vi "ClimbSequencer.vi"(7 "Reinit":bool) -> (0 "Climber Climbing":bool, 1 "Climber Power":dbl, 2 "Climber Pin":bool, 3 "PTO":bool)   [LabVIEW 2019]
doc: "This VI contains the endgame climb sequencer."
uses:
  dscommands.vi
  78443452-49a0-4252-95b8-0a958b59513b.vi
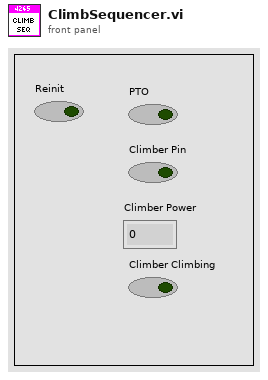
[diagram p1: front panel]
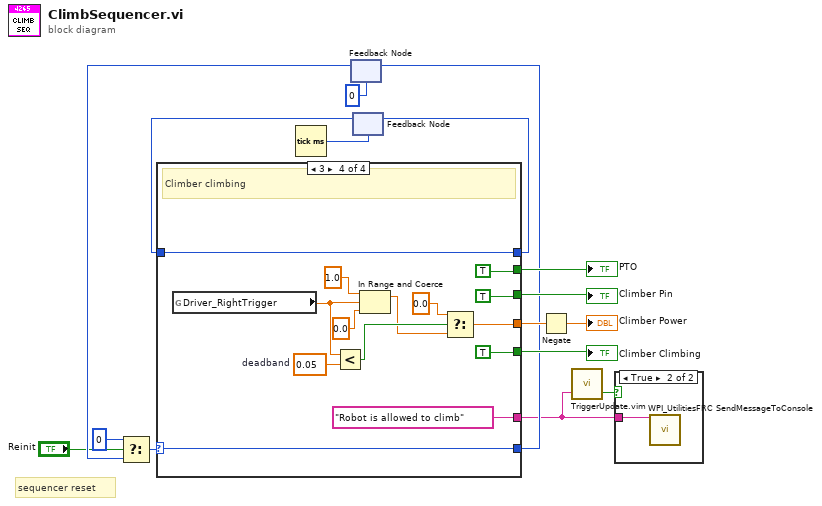
[diagram p0: block diagram]
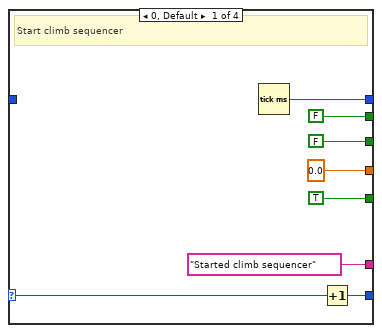
[diagram p3: hidden frame]
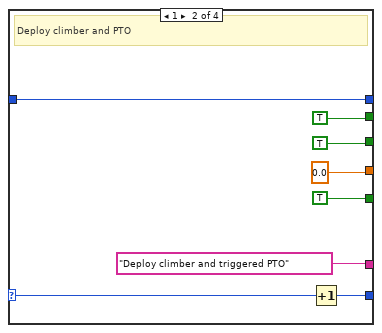
[diagram p4: hidden frame]
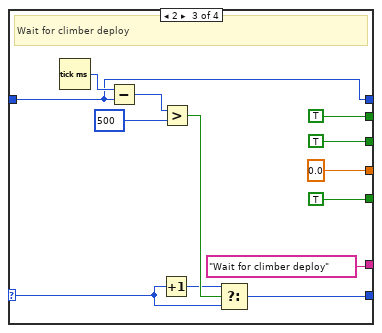
[diagram p5: hidden frame]
diagram:
  # "sequencer reset"
  n1 = Tick Count (ms)() -> (millisecond timer value=w7:u32)
  n2 = feedback #1(0) -> (w13:i32)
  n3 = Select(t=0, s="Reinit", f=w13) -> (s? t:f=w15:i32)
  n4 = feedback #2(w7) -> (w6:u32)
  n5 = case shown="3" w15 {
    selector: w15 -> [w22 w32 w41 w58]
    tunnel: [w21 w27 w39 w58] -> w3
    tunnel: ["Started climb sequencer" "Deploy climber and triggered PTO" "Wait for climber deploy" "Robot is allowed to climb"] -> w2
    tunnel: [w24 w28 w38 w57] -> w5
    tunnel: w6 -> [_ w28 w38 w57]
    tunnel: [0.0 ("Climber_Power") 0.0 ("Climber_Power") 0.0 ("Climber_Power") w53] -> w8
    tunnel: [FALSE TRUE TRUE TRUE] -> w9
    tunnel: [FALSE TRUE TRUE TRUE] -> w10
    tunnel: [TRUE TRUE TRUE TRUE] -> w11
    frame 0, Default {
      # "Start climb sequencer"
      n6 = Tick Count (ms)() -> (millisecond timer value=w24:u32)
      n7 = Increment(x=w22) -> (x+1=w21:i32)
    }
    frame 1 {
      # "Deploy climber and PTO"
      n8 = Increment(x=w32) -> (x+1=w27:i32)
    }
    frame 2 {
      # "Wait for climber deploy"
      n9 = Tick Count (ms)() -> (millisecond timer value=w45:u32)
      n10 = Subtract(x=w45, y=w38) -> (x-y=w44:u32)
      n11 = Increment(x=w41) -> (x+1=w40:i32)
      n12 = Greater?(x=w44, y=u32 500) -> (0:w42:bool)
      n13 = Select(t=w40, s=w42, f=w41) -> (s? t:f=w39:i32)
    }
    frame 3 {
      w50 = 0.05  # deadband
      # "Climber climbing"
      n14 = global read "dscommands.vi" "Driver_RightTrigger"() -> (w46:dbl)
      n15 = Less?(x=w46, y=w50) -> (x < y?=w52:bool)
      n16 = In Range and Coerce(upper limit=1.0, x=w46, lower limit=0.0) -> (coerced(x)=w49:dbl)  [unwired: 1 out]
      n17 = Select(t=0.0, s=w52, f=w49) -> (s? t:f=w53:dbl)
    }
  }
  "Climber Climbing" <- w11
  "Climber Pin" <- w10
  "PTO" <- w9
  n18 = feedback-in #1(w3) -> ()
  n19 = feedback-in #2(w5) -> ()
  n20 = Negate(x=w8) -> (-x=→"Climber Power":dbl)
  n21 = call "TriggerUpdate.vim"("Trigger"=w2) -> ("Update"=w1:bool)  [unwired: 2 in]
  n22 = case shown="True" w1 {
    tunnel: w2 -> [_ w60]
    frame False {
    }
    frame True {
      n23 = call <vilib>:"WPI_UtilitiesFRC SendMessageToConsole.vi"("Message"=w60) -> ()  [unwired: 14 in, 1 out]
    }
  }
